vi "Get Type Description.vi"(8 "error in (no error)":errorcluster, 11 "Step in":refnum<class "Step.lvclass">) -> (0 "error out":errorcluster, 2 "Type Description":string, 3 "Step out":refnum<class "Step.lvclass">)   [LabVIEW 2020, in "MacroAssert.lvlib" / "Step.lvclass"]
uses:
  Step.lvclass
  Step.lvclass/Step.ctl
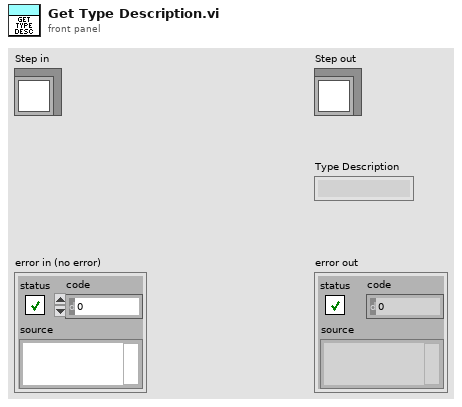
[diagram p1: front panel]
types:
  T1 = typedef "MacroAssert.lvlib/Step Type V3.ctl" = enum16{"Mouse Action", "Keyboard Action", "Window Action", "Timing Action", "Boolean Assertion", "Numeric Assertion", "String Assertion", "Image Assertion"}
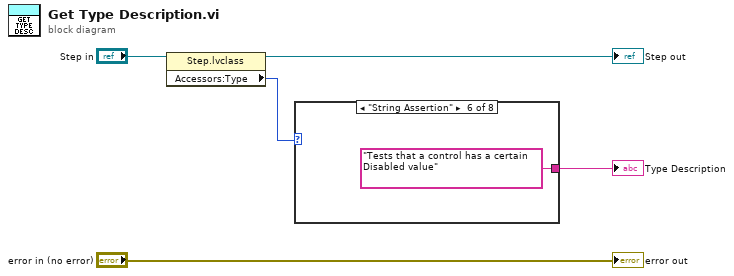
[diagram p0: block diagram]
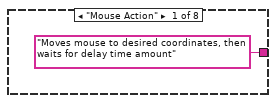
[diagram p2: hidden frame]
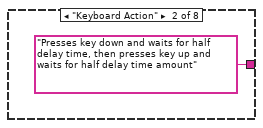
[diagram p3: hidden frame]
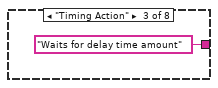
[diagram p4: hidden frame]
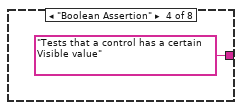
[diagram p5: hidden frame]
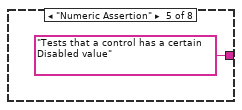
[diagram p6: hidden frame]
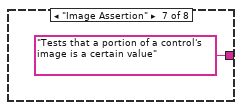
[diagram p7: hidden frame]
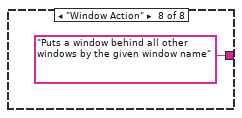
[diagram p8: hidden frame]
diagram:
  n1 = property class="Step.lvclass"(reference="Step in") -> (reference out=→"Step out":refnum<class "Step.lvclass">, "Accessors:Type"=w2:T1)  [unwired: 1 in, 1 out]
  n2 = case shown="\"String Assertion\"" w2 {
    tunnel: ["Moves mouse to desired coordinates, then waits for delay time amount" "Presses key down and waits for half delay time, then presses key up and waits for half delay time amount" "Waits for delay time amount" "Tests that a control has a certain Visible value" "Tests that a control has a certain Disabled value" "Tests that a control has a certain Disabled value" "Tests that a portion of a control's image is a certain value" "Puts a window behind all other windows by the given window name"] -> w1
    frame "Mouse Action" {
    }
    frame "Keyboard Action" {
    }
    frame "Timing Action" {
    }
    frame "Boolean Assertion" {
    }
    frame "Numeric Assertion" {
    }
    frame "String Assertion" {
    }
    frame "Image Assertion" {
    }
    frame "Window Action" {
    }
  }
  "Type Description" <- w1
  "error out" <- "error in (no error)"
